vi "_snippet_.vi"   [LabVIEW 2019]
uses:
  VsDebugLibrary.lvlib
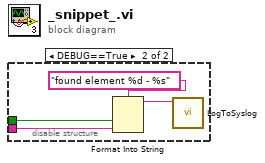
[diagram p0: block diagram]
diagram:
  n1 = disable-structure shown="DEBUG==True" {
    disable-tunnel: _ -> [_ w3]
    disable-tunnel: _ -> [_ w4]
    frame condition #0 {
    }
    frame condition #1 (active) {
      n2 = Format Into String(format string="found element %d - %s", w3, w4) -> (resulting string=w1:string)  [unwired: 2 in, 1 out]
      n3 = call "LogToSyslog.vi"("message"=w1) -> ()  [unwired: 9 in, 2 out]
    }
  }
